vi "receiveData.vi"(8 "error in (no error)":errorcluster, 11 "Model in":refnum<class "Model.lvclass">) -> (0 "error out":errorcluster, 3 "Model out":refnum<class "Model.lvclass">)   [LabVIEW 2015, in "Model.lvclass"]
uses:
  Model.lvclass
  Model.lvclass/Model.ctl
  <userlib>/Common/ILC/ILC/ILC.lvclass/ILC.ctl
  <userlib>/Common/ILC/ILC/ILC.lvclass
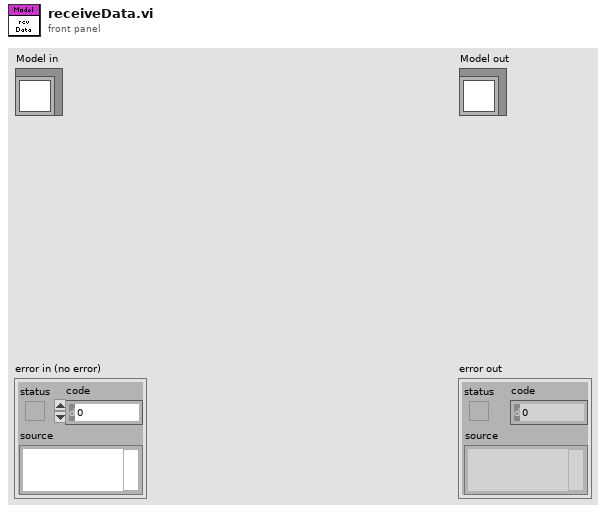
[diagram p1: front panel]
types:
  T1 = typedef "ILCCommon.lvlib/ILCTypedefs.lvlib/InputData.ctl" = cluster{"Input Channels":T2, "Limit Switches":T3, "Tachometer":u16, "SSI Encoder":i32, "ADCs":T4}
  T2 = typedef "ILCCommon.lvlib/ILCConfiguration.lvlib/InputChannels.ctl" = enum16{"Channel 0", "3 Channels", "5 Channels"}
  T3 = typedef "ILCCommon.lvlib/ILCTypedefs.lvlib/LimitSwitches.ctl" = cluster{"1":bool, "2":bool}
  T4 = typedef "ILCCommon.lvlib/ILCTypedefs.lvlib/ADCs.ctl" = cluster{"Ch0":i32, "Ch1":i32, "Ch2":i32, "Ch3":i32, "Ch4":i32}
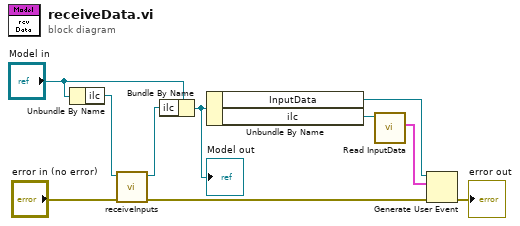
[diagram p0: block diagram]
diagram:
  n1 = Unbundle By Name("Model in") -> ("ilc"=w4:refnum<class "ILC.lvclass">)
  n2 = call <userlib>:"receiveInputs.vi"("error in (no error)"="error in (no error)", "ILC in"=w4) -> ("error out"=w1:errorcluster, "ILC out"=w3:refnum<class "ILC.lvclass">)  [unwired: 6 in, 2 out]
  n3 = Bundle By Name(cluster="Model in", "ilc"=w3) -> (w5:refnum<class "Model.lvclass">)
  "Model out" <- w5
  n4 = Unbundle By Name(w5) -> ("InputData"=w10:refnum<user-event>, "ilc"=w8:refnum<class "ILC.lvclass">)
  n5 = call <userlib>:"Read InputData.vi"("ILC in"=w8) -> ("InputData"=w7:T1)  [unwired: 9 in, 1 out]
  n6 = Generate User Event(user event=w10, event data cluster=w7, error in=w1) -> (error out=→"error out":errorcluster)  [unwired: 1 in, 1 out]
